vi "Init.vi"(8 "error in (no error)":errorcluster, 10 "Default Index File (index.html)":string="index.html", 11 "Public Root":path) -> (0 "error out":errorcluster, 3 "TemplatedFileServe out":refnum<class "TemplatedFileServe.lvclass">)   [LabVIEW 2020, in "HTTP Server.lvlib" / "TemplatedFileServe.lvclass"]
uses:
  TemplatedFileServe.lvclass
  TemplatedFileServe.lvclass/TemplatedFileServe.ctl
  StandardFileServe/StandardFileServe.lvclass
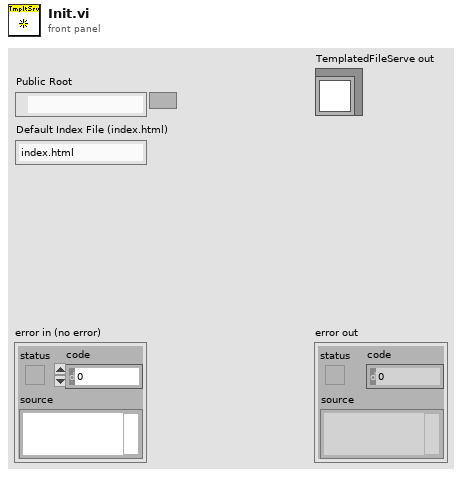
[diagram p1: front panel]
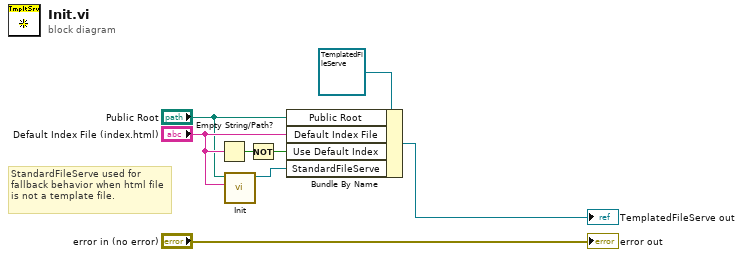
[diagram p0: block diagram]
diagram:
  # "StandardFileServe used for fallback behavior when html file is not a template file."
  n1 = Empty String/Path?(string/path="Default Index File (index.html)") -> (empty?=w5:bool)
  n2 = call "Init.vi"("Default Index File (index.html)"="Default Index File (index.html)", "Public Root"="Public Root") -> ("StandardFileServe out"=w1:refnum<class "StandardFileServe.lvclass">)  [unwired: 8 in, 1 out]
  n3 = Not(x=w5) -> (.not. x?=w4:bool)
  n4 = Bundle By Name(cluster=refnum<class "TemplatedFileServe.lvclass"> refnum ("TemplatedFileServe in"), "Public Root"="Public Root", "Default Index File"="Default Index File (index.html)", "Use Default Index"=w4, "StandardFileServe"=w1) -> (→"TemplatedFileServe out":refnum<class "TemplatedFileServe.lvclass">)
  "error out" <- "error in (no error)"
